vi "Read Logical Instrument.vi"(8 "error in (no error)":errorcluster, 11 "Instrument in":refnum<class "Instrument.lvclass">) -> (0 "error out":errorcluster, 2 "Logical Instrument":string, 3 "Instrument out":refnum<class "Instrument.lvclass">)   [LabVIEW 2023, in "HAF.lvlib" / "Instrument.lvclass"]
uses:
  Instrument.lvclass
  Instrument.lvclass/Instrument.ctl
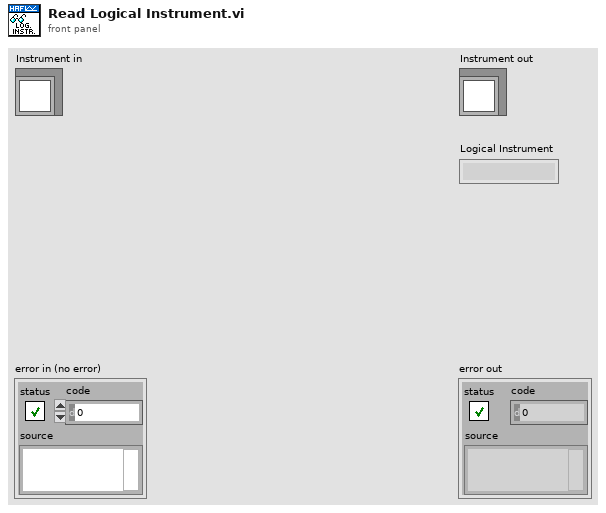
[diagram p1: front panel]
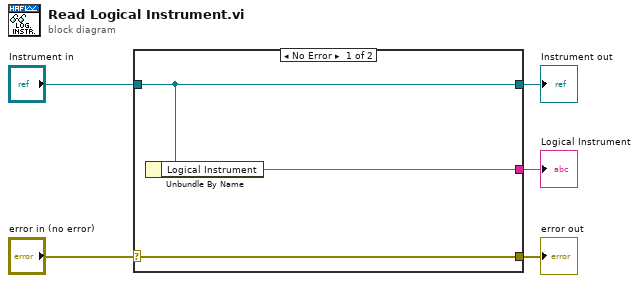
[diagram p0: block diagram]
diagram:
  n1 = case shown="No Error" "error in (no error)" {
    selector: "error in (no error)" -> [w8 w9]
    tunnel: [w8 w9] -> w4
    tunnel: [w7 w10] -> w2
    tunnel: "Instrument in" -> [w7 w10]
    tunnel: [w6 _] -> w1
    frame No Error {
      n2 = Unbundle By Name(w7) -> ("Logical Instrument"=w6:string)
    }
    frame Error {
    }
  }
  "error out" <- w4
  "Instrument out" <- w2
  "Logical Instrument" <- w1
